vi "subFinalize HW (niUSRP).vi"(0 "Tx Settings":T1={"USRP IP Address"="192.168.11.4", "IQ Sampling\nRate [S/sec]"=10000000.0, "Carrier Frequency [Hz]"=87000000.0, "Start Trigger Time"={"whole seconds"=0, "fractional seconds"=0.0}, "Per Device"=[]} {"Per Device"."gain" format="%#_6f"; "Carrier Frequency [Hz]" min=50000000.0 max=6000000000.0 step=1000.0 format="%#.15p"; "IQ Sampling\nRate [S/sec]" format="%#_6p"}, 5 "Rx Settings":T1={"USRP IP Address"="192.168.11.4", "IQ Sampling\nRate [S/sec]"=10000000.0, "Carrier Frequency [Hz]"=87000000.0, "Start Trigger Time"={"whole seconds"=0, "fractional seconds"=0.0}, "Per Device"=[]} {"Per Device"."gain" format="%#_6f"; "Carrier Frequency [Hz]" min=50000000.0 max=6000000000.0 step=1000.0 format="%#.15p"; "IQ Sampling\nRate [S/sec]" format="%#_6p"}, 11 "error in (no error)":errorcluster) -> (15 "error out":errorcluster)   [LabVIEW 2011]
uses:
  usrpHardwareSettings.ctl
  <instrlib>/niUSRP/niUSRP Timestamp.ctl
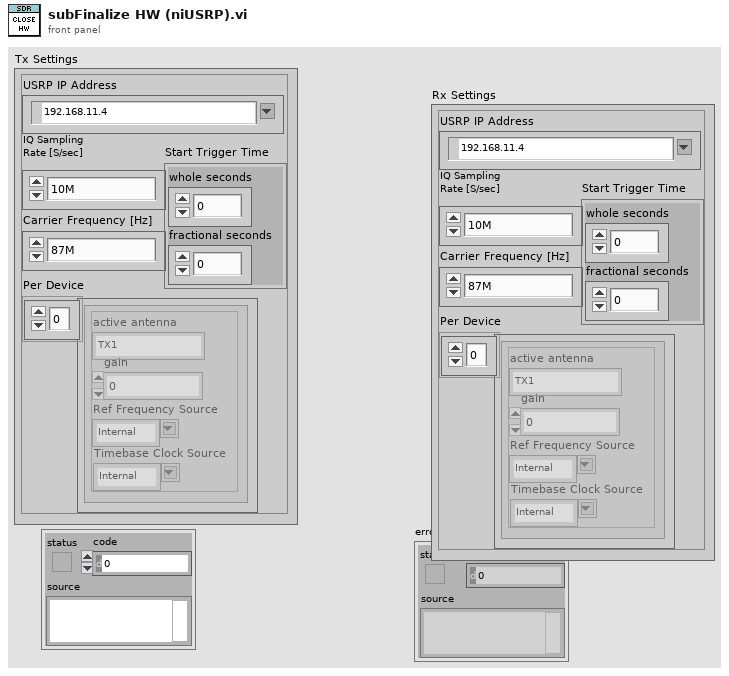
[diagram p1: front panel]
types:
  T1 = typedef "usrpHardwareSettings.ctl" = cluster{"USRP IP Address":refnum<k15>, "IQ Sampling\nRate [S/sec]":dbl, "Carrier Frequency [Hz]":dbl, "Start Trigger Time":T2, "Per Device":cluster{"active antenna":string, "gain":dbl, "Ref Frequency Source":string, "Timebase Clock Source":string}[]}
  T2 = typedef "niUSRP Timestamp.ctl" = cluster{"whole seconds":u64, "fractional seconds":dbl}
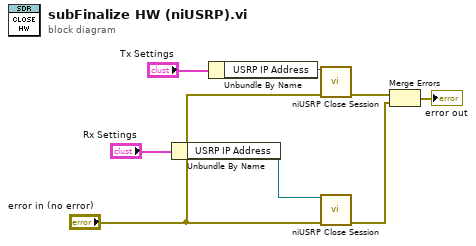
[diagram p0: block diagram]
diagram:
  n1 = Unbundle By Name("Rx Settings") -> ("USRP IP Address"=w2:refnum<k15>)
  n2 = Unbundle By Name("Tx Settings") -> ("USRP IP Address"=w1:refnum<k15>)
  n3 = call <instrlib>:"niUSRP Close Session.vi"("session handle"=w1, "error in (no error)"="error in (no error)") -> ("error out"=w6:errorcluster)  [unwired: 13 in]
  n4 = call <instrlib>:"niUSRP Close Session.vi"("session handle"=w2, "error in (no error)"="error in (no error)") -> ("error out"=w5:errorcluster)  [unwired: 13 in]
  n5 = Merge Errors(w6, w5) -> (→"error out":errorcluster)
